vi "brakecontrol1.vi"(8 "e-stop":bool, 10 "theta_encoder":dbl=-3.279271506191265, 11 "theta_des":dbl=0.2849002849002849) -> (3 "Tm_ff[duty%]":dbl=2.2396851483757043)   [LabVIEW 2012]
panel:
  out "Waveform Chart 2":dbl(graph)
  in  "tuning_gain2 2":dbl=0.5
  in  "Boolean 2":bool=TRUE
  out "Waveform Chart":dynamicdata(graph)=[{"t0"=timestamp(3412698537.013247 s since 1904-01-01), "dt"=1.0, "Y"=[0.2849002849002849]}, {"t0"=timestamp(3412698537.0131693 s since 1904-01-01), "dt"=1.0, "Y"=[-3.279271506191265]}]
  in  "gain":dbl=7.0
  in  "Boolean":bool=TRUE
  out "theta_vel_des":dbl
  in  "FBGain":dbl=1.0
  in  "P_gain":dbl=4.0
  in  "D_gain":dbl=0.05
  in  "FFGain":dbl=0.02
  in  "ICG":dbl=0.035
  in  "g":dbl=9.81
  in  "m":dbl=1.0
  in  "thetaCG":dbl=5.0
  in  "b":dbl=20.0
  in  "mu_visc":dbl=0.01
  in  "mu_coul":dbl=0.19
  in  "gain20":dbl=1000.0
  in  "gain4":dbl=1.0
  in  "gain3":dbl=1.0
  in  "gain2":dbl=0.5
  in  "tuning_gain2":dbl=1.0
  in  "tuning_gain1":dbl
  in  "lc":dbl=1.5
  out "theta_acc_des":dbl
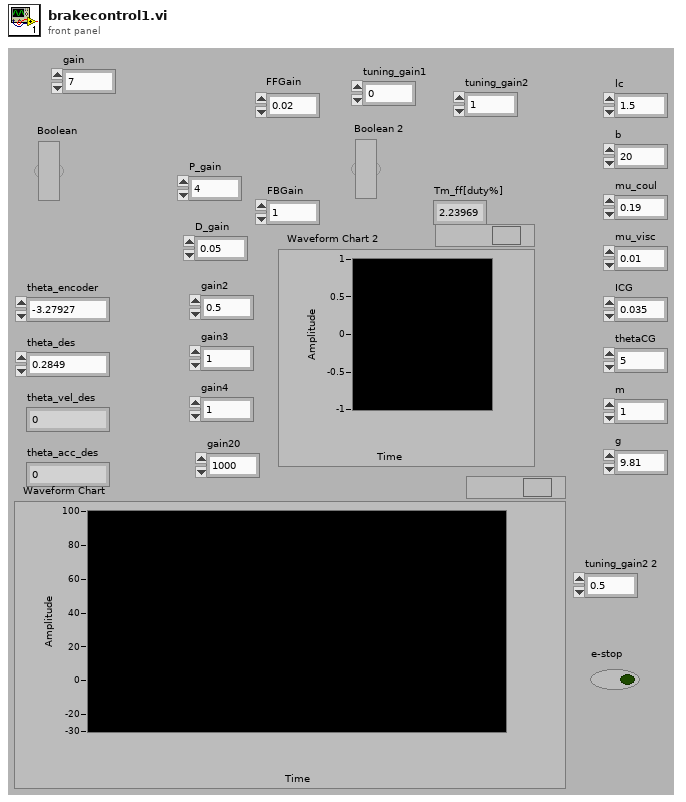
[diagram p1: front panel]
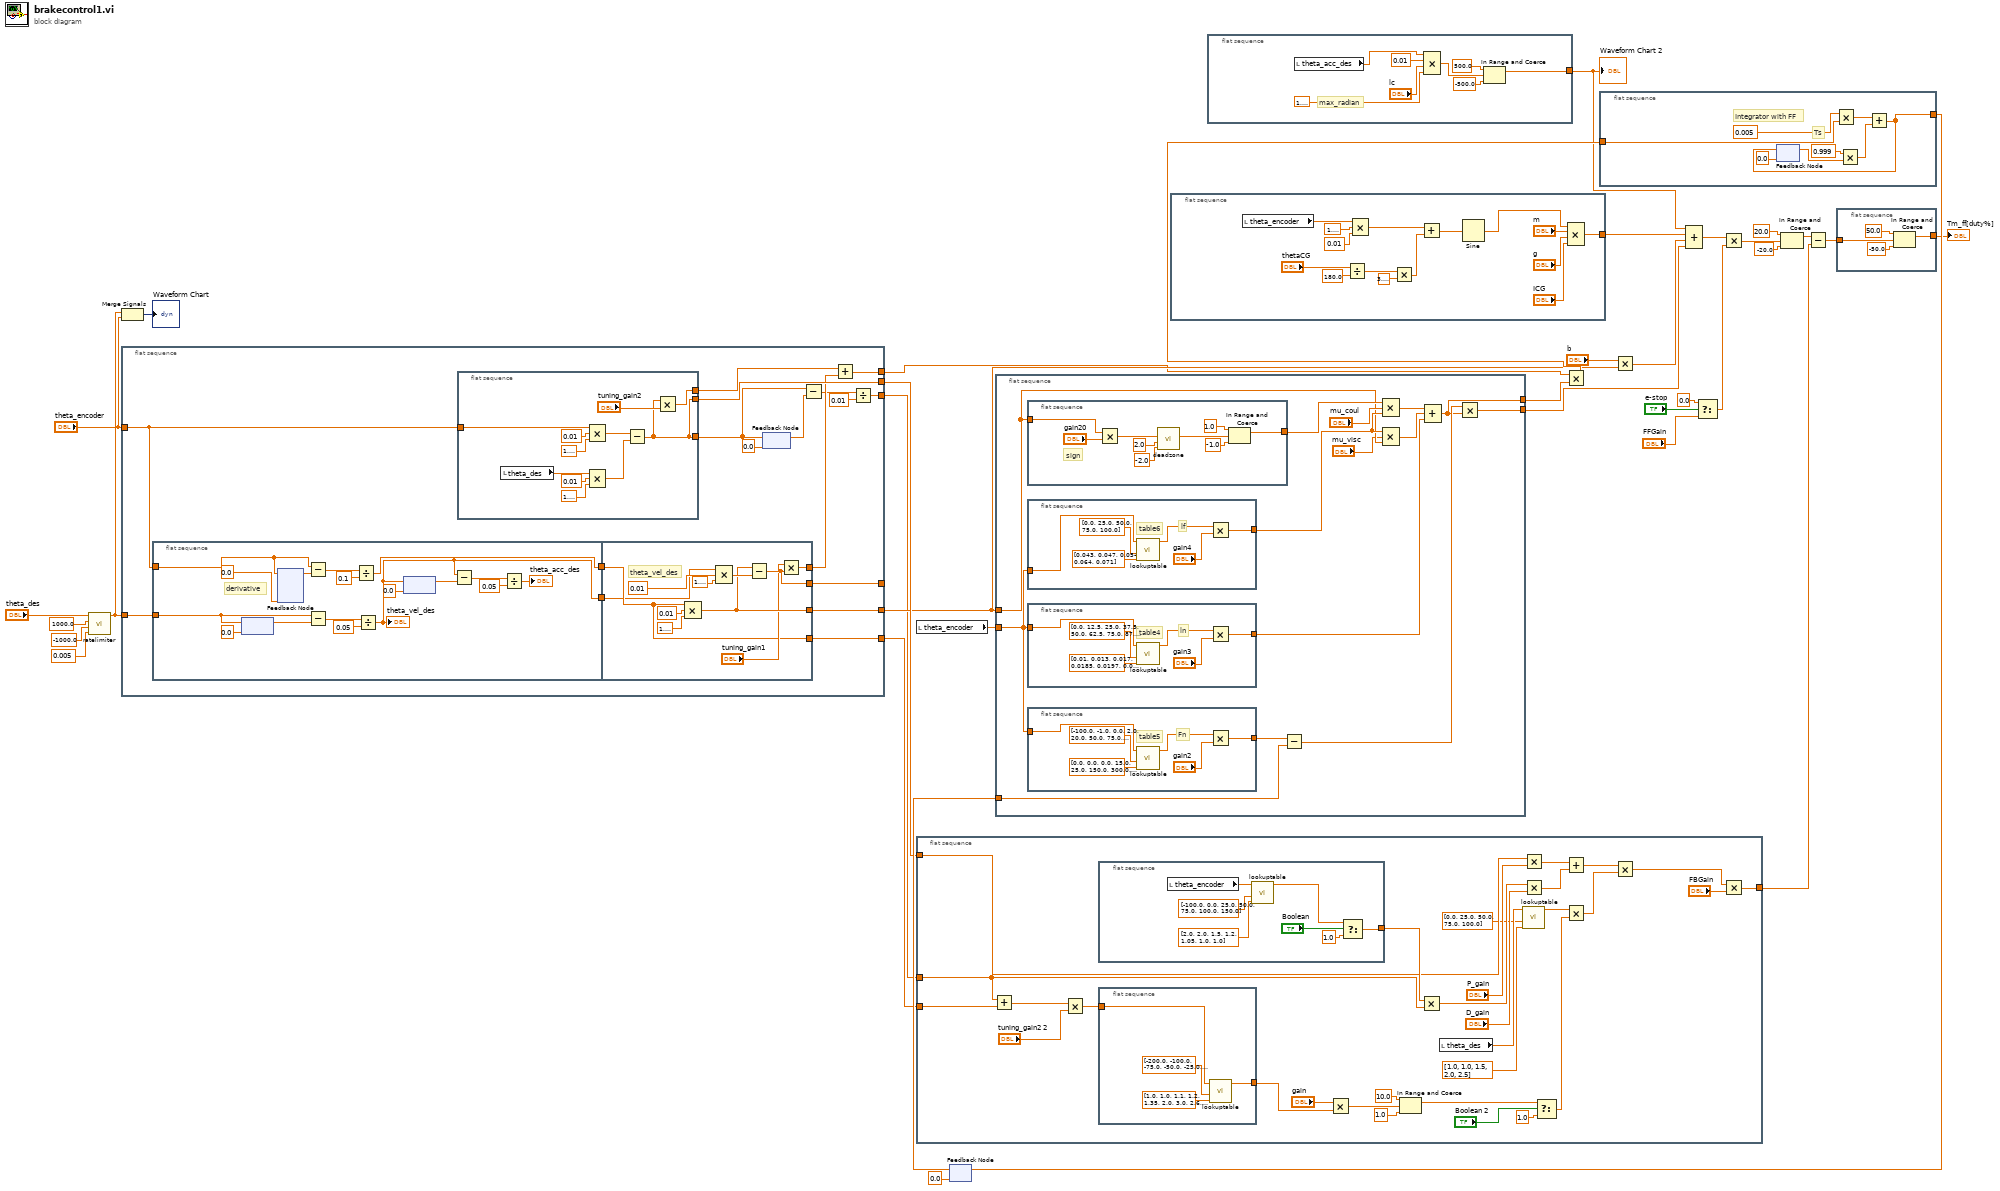
[diagram p0: block diagram]
diagram:
  n1 = call "ratelimiter.vi"("Ts"=0.005, "falling slew rate"=-1000.0, "rising slew rate"=1000.0, "input"="theta_des") -> ("output"=w15:dbl)  [unwired: 6 in, 1 out]
  n2 = Merge Signals(w15, "theta_encoder") -> (→"Waveform Chart":dynamicdata)
  n3 = flat-sequence {
    tunnel: [w52] -> w9
    tunnel: "theta_encoder" -> [w49]
    tunnel: [w51] -> w22
    tunnel: [w48] -> _
    tunnel: [w47] -> w27
    tunnel: [w46] -> w26
    tunnel: w15 -> [w44]
    tunnel: [w36] -> w11
    frame #0 {
      n4 = flat-sequence {
        tunnel: w49 -> [w79]
        tunnel: [w76] -> w50
        tunnel: [w64] -> w45
        tunnel: w44 -> [w67]
        tunnel: [w88] -> w43
        tunnel: [w85] -> w51
        tunnel: w50 -> [w82]
        tunnel: [w84] -> w48
        tunnel: [w82] -> w46
        tunnel: w45 -> [w81]
        frame #0 {
          # "derivative"
          n5 = feedback #1(0.0 ("input")) -> (w69:dbl)
          n6 = feedback-in #1(w67) -> ()
          n7 = feedback #2(0.0 ("input")) -> (w78:dbl)
          n8 = feedback-in #2(w79) -> ()
          n9 = Subtract(x=w79, y=w78) -> (x-y=w74:dbl)
          n10 = Subtract(x=w67, y=w69) -> (x-y=w66:dbl)
          n11 = Divide(x=w74, y=0.1) -> (x/y=w76:dbl)
          n12 = Divide(x=w66, y=0.05) -> (x/y=w64:dbl)
          "theta_vel_des" <- w64
          n13 = feedback #3(0.0 ("input")) -> (w73:dbl)
          n14 = feedback-in #3(w64) -> ()
          n15 = Subtract(x=w64, y=w73) -> (x-y=w71:dbl)
          n16 = Divide(x=w71, y=0.05) -> (x/y=→"theta_acc_des":dbl)
        }
        frame #1 {
          # "theta_vel_des"
          n17 = Compound Arithmetic op=MULTIPLY(w82, 0.01 ("value"), 1.5707963267948966) -> (w85:dbl)
          n18 = Compound Arithmetic op=MULTIPLY(w81, 0.01 ("value"), 1.5707963267948966) -> (w89:dbl)
          n19 = Subtract(x=w85, y=w89) -> (x-y=w84:dbl)
          n20 = Multiply(x="tuning_gain1", y=w84) -> (x*y=w88:dbl)
        }
      }
      n21 = flat-sequence {
        tunnel: w49 -> [w62]
        tunnel: [w61] -> w42
        tunnel: [w53] -> w47
        tunnel: [w53] -> w37
        frame #0 {
          n22 = local read "theta_des"() -> (w54:dbl)
          n23 = Compound Arithmetic op=MULTIPLY(w62, 0.01 ("value"), 1.5707963267948966) -> (w63:dbl)
          n24 = Compound Arithmetic op=MULTIPLY(w54, 0.01 ("value"), 1.5707963267948966) -> (w56:dbl)
          n25 = Subtract(x=w63, y=w56) -> (x-y=w53:dbl)
          n26 = Multiply(x=w53, y="tuning_gain2") -> (x*y=w61:dbl)
        }
      }
      n27 = feedback #4(0.0 ("input")) -> (w39:dbl)
      n28 = feedback-in #4(w37) -> ()
      n29 = Subtract(x=w37, y=w39) -> (x-y=w41:dbl)
      n30 = Add(x=w42, y=w43) -> (x+y=w52:dbl)
      n31 = Divide(x=w41, y=0.01) -> (x/y=w36:dbl)
    }
  }
  n32 = local read "theta_encoder"() -> (w32:dbl)
  n33 = flat-sequence {
    tunnel: w11 -> [w105]
    tunnel: w27 -> [w118]
    tunnel: w26 -> [w106]
    tunnel: [w114] -> w25
    frame #0 {
      n34 = Add(x=w105, y=w106) -> (x+y=w103:dbl)
      n35 = Multiply(x=w103, y="tuning_gain2 2") -> (x*y=w102:dbl)
      n36 = flat-sequence {
        tunnel: [w127] -> w121
        frame #0 {
          n37 = local read "theta_encoder"() -> (w132:dbl)
          n38 = call "lookuptable.vi"("array_y"=dbl[] [2.0, 2.0, 1.5, 1.2, 1.05, 1.0, 1.0] ("array_x"), "array_x"=dbl[] [-100.0, 0.0, 25.0, 50.0, 75.0, 100.0, 150.0], "x"=w132) -> ("y"=w128:dbl)  [unwired: 8 in]
          n39 = Select(t=w128, s="Boolean", f=1.0) -> (s? t:f=w127:dbl)
        }
      }
      n40 = flat-sequence {
        tunnel: w102 -> [w123]
        tunnel: [w122] -> w109
        frame #0 {
          n41 = call "lookuptable.vi"("array_y"=dbl[] [1.0, 1.0, 1.1, 1.2, 1.35, 2.0, 3.0, 2.6, 2.3, 2.1, 2.0, 2.0] ("array_x"), "array_x"=dbl[] [-200.0, -100.0, -75.0, -50.0, -25.0, -1.0, 0.0, 25.0, 50.0, 75.0, 100.0, 200.0], "x"=w123) -> ("y"=w122:dbl)  [unwired: 8 in]
        }
      }
      n42 = Multiply(x="gain", y=w109) -> (x*y=w93:dbl)
      n43 = In Range and Coerce(upper limit=10.0 ("max"), x=w93, lower limit=1.0 ("min")) -> (coerced(x)=w92:dbl)  [unwired: 1 out]
      n44 = Multiply(x=w121, y=w105) -> (x*y=w120:dbl)
      n45 = local read "theta_des"() -> (w99:dbl)
      n46 = call "lookuptable.vi"("array_y"=dbl[] [1.0, 1.0, 1.5, 2.0, 2.5] ("array_x"), "array_x"=dbl[] [0.0, 25.0, 50.0, 75.0, 100.0], "x"=w99) -> ("y"=w98:dbl)  [unwired: 8 in]
      n47 = Multiply(x=w118, y="P_gain") -> (x*y=w111:dbl)
      n48 = Multiply(x=w120, y="D_gain") -> (x*y=w112:dbl)
      n49 = Select(t=w92, s="Boolean 2", f=1.0) -> (s? t:f=w101:dbl)
      n50 = Add(x=w111, y=w112) -> (x+y=w113:dbl)
      n51 = Multiply(x=w98, y=w101) -> (x*y=w100:dbl)
      n52 = Multiply(x=w113, y=w100) -> (x*y=w116:dbl)
      n53 = Multiply(x=w116, y="FBGain") -> (x*y=w114:dbl)
    }
  }
  n54 = feedback #5(0.0 ("input")) -> (w28:dbl)
  n55 = feedback-in #5(w34) -> ()
  n56 = flat-sequence {
    tunnel: w22 -> [w142]
    tunnel: [w133] -> w20
    tunnel: [w138] -> w29
    tunnel: w28 -> [w136]
    tunnel: w32 -> [w135]
    frame #0 {
      n57 = flat-sequence {
        tunnel: w142 -> [w173]
        tunnel: [w165] -> w145
        frame #0 {
          # "sign"
          n58 = Multiply(x=w173, y="gain20") -> (x*y=w171:dbl)
          n59 = call "deadzone.vi"("min"=-2.0, "max"=2.0, "x"=w171) -> ("dead zone"=w168:dbl)  [unwired: 8 in]
          n60 = In Range and Coerce(upper limit=1.0 ("max"), x=w168, lower limit=-1.0 ("min")) -> (coerced(x)=w165:dbl)  [unwired: 1 out]
        }
      }
      n61 = flat-sequence {
        tunnel: w135 -> [w162]
        tunnel: [w159] -> w143
        frame #0 {
          # "lf"
          # "table6"
          n62 = call "lookuptable.vi"("array_y"=dbl[] [0.043, 0.047, 0.054, 0.064, 0.071], "array_x"=dbl[] [0.0, 25.0, 50.0, 75.0, 100.0], "x"=w162) -> ("y"=w160:dbl)  [unwired: 8 in]
          n63 = Multiply(x=w160, y="gain4") -> (x*y=w159:dbl)
        }
      }
      n64 = flat-sequence {
        tunnel: w135 -> [w155]
        tunnel: [w153] -> w139
        frame #0 {
          # "ln"
          # "table4"
          n65 = call "lookuptable.vi"("array_y"=dbl[] [0.01, 0.013, 0.017, 0.0185, 0.0197, 0.02, 0.193, 0.017, 0.012], "array_x"=dbl[] [0.0, 12.5, 25.0, 37.5, 50.0, 62.5, 75.0, 87.5, 100.0], "x"=w155) -> ("y"=w154:dbl)  [unwired: 8 in]
          n66 = Multiply(x=w154, y="gain3") -> (x*y=w153:dbl)
        }
      }
      n67 = flat-sequence {
        tunnel: [w148] -> w146
        tunnel: w135 -> [w147]
        frame #0 {
          # "Fn"
          # "table5"
          n68 = call "lookuptable.vi"("array_y"=dbl[] [0.0, 0.0, 0.0, 15.0, 25.0, 150.0, 300.0, 930.0], "array_x"=dbl[] [-100.0, -1.0, 0.0, 2.0, 20.0, 50.0, 75.0, 100.0], "x"=w147) -> ("y"=w150:dbl)  [unwired: 8 in]
          n69 = Multiply(x=w150, y="gain2") -> (x*y=w148:dbl)
        }
      }
      n70 = Subtract(x=w146, y=w136) -> (x-y=w134:dbl)
      n71 = Compound Arithmetic op=MULTIPLY(w145, "mu_coul", w143) -> (w141:dbl)
      n72 = Compound Arithmetic op=MULTIPLY(w143, "mu_visc", w142) -> (w140:dbl)
      n73 = Compound Arithmetic op=ADD(w141, w140, w139) -> (w133:dbl)
      n74 = Multiply(x=w134, y=w133) -> (x*y=w138:dbl)
    }
  }
  n75 = flat-sequence {
    tunnel: [w178] -> w21
    frame #0 {
      n76 = local read "theta_encoder"() -> (w177:dbl)
      n77 = Divide(x="thetaCG", y=180.0) -> (x/y=w186:dbl)
      n78 = Compound Arithmetic op=MULTIPLY(w177, 1.5707963267948966, 0.01 ("value")) -> (w174:dbl)
      n79 = Multiply(x=w186, y=3.141592653589793) -> (x*y=w184:dbl)
      n80 = Add(x=w174, y=w184) -> (x+y=w183:dbl)
      n81 = Sine(x=w183) -> (sin(x)=w182:dbl)
      n82 = Compound Arithmetic op=MULTIPLY(w182, "m", "g", "ICG") -> (w178:dbl)
    }
  }
  n83 = flat-sequence {
    tunnel: [w189] -> w12
    frame #0 {
      # "max_radian"
      n84 = local read "theta_acc_des"() -> (w193:dbl)
      n85 = Compound Arithmetic op=MULTIPLY(w193, 0.01 ("value"), "lc", 1.5707963267948966) -> (w190:dbl)
      n86 = In Range and Coerce(upper limit=500.0 ("max"), x=w190, lower limit=-500.0 ("min")) -> (coerced(x)=w189:dbl)  [unwired: 1 out]
    }
  }
  n87 = Multiply(x=w9, y=w20) -> (x*y=w35:dbl)
  n88 = flat-sequence {
    tunnel: w35 -> [w198]
    tunnel: [w197] -> w34
    frame #0 {
      # "Integrator with FF"
      # "Ts"
      n89 = feedback #6(0.0 ("input")) -> (w200:dbl)
      n90 = Multiply(x=0.005 ("Ts"), y=w198) -> (x*y=w204:dbl)
      n91 = Multiply(x=0.999, y=w200) -> (x*y=w201:dbl)
      n92 = Add(x=w204, y=w201) -> (x+y=w197:dbl)
      n93 = feedback-in #6(w197) -> ()
    }
  }
  n94 = Multiply(x="b", y=w22) -> (x*y=w24:dbl)
  n95 = Compound Arithmetic op=ADD(w12, w21, w24, w29) -> (w31:dbl)
  n96 = Select(t=0.0, s="e-stop", f="FFGain") -> (s? t:f=w5:dbl)
  n97 = Multiply(x=w31, y=w5) -> (x*y=w2:dbl)
  n98 = In Range and Coerce(upper limit=20.0 ("max"), x=w2, lower limit=-20.0 ("min")) -> (coerced(x)=w1:dbl)  [unwired: 1 out]
  n99 = Subtract(x=w1, y=w25) -> (x-y=w30:dbl)
  n100 = flat-sequence {
    tunnel: w30 -> [w208]
    tunnel: [w205] -> w10
    frame #0 {
      n101 = In Range and Coerce(upper limit=50.0 ("max"), x=w208, lower limit=-50.0 ("min")) -> (coerced(x)=w205:dbl)  [unwired: 1 out]
    }
  }
  "Tm_ff[duty%]" <- w10
  "Waveform Chart 2" <- w12
